vi "Compute 1-Exp Gate Array v2.vi"(8 "Error In":errorcluster, 9 "Gates Definitions":T3={"First Gate: t1"=0.0, "Gate Width: W"=0.0, "Gate Step: d"=0.0, "# Gates: G"=0.0, "Use Gate Center"=FALSE, "Frames/Image: F"=50, "Gates/Frame: L"=0, "Bits/Frame: q"=0, "Multiplicity: p"=0, "Gate Type"=enum."Square", "Gate Edge s"=4.0, "Gate Top Slope"=4.0, "Reversed Sawtooth?"=FALSE, "Computation"=FALSE, "User-defined Gate"={"X Array"=[], "Y Array"=[]}, "Tolerance"=50.0, "Integration"=enum."Item 0", "# Steps"=50.0, "Type of User-defined Function"=enum."Gate"}, 11 "Decay Definition":T1={"offset: t0"=0.0, "period: T"=0.0, "lifetime: tau"=0.0, "Incident Signal: I"=0.5, "Normalized Decays"=FALSE, "IRF Model"=enum."Dirac", "IRF Parameter 1"=0.0}) -> (0 "Error Out":errorcluster, 1 "Gate Image Array":ext[](array[numeric]), 3 "t Array":ext[](array[numeric]), 4 "Small Gate Values?":bool, 6 "CPU (s)":dbl)   [LabVIEW 2019]
uses:
  Gate Definitions.ctl
  Gate Type.ctl
  XY Plot Data.ctl
  Decay Definiton.ctl
  IRF Model.ctl
  Photon-Counting Saturation Parameters.ctl
  Linear Ramp End Options.ctl
  Gate & Decay Parameters.ctl
  <vilib>/Analysis/2dsp.llb/Integral Method.ctl
  <vilib>/Utility/High Resolution Relative Seconds.vi
  9dc9122e-8396-4e29-9b52-206296392f6e.vi/00547001-b378-40f2-b110-93d9ac793ed4.vi
  9dc9122e-8396-4e29-9b52-206296392f6e.vi/724eff8e-639b-48e4-a8a7-ae0679ec3008.vi
  09e65239-3f09-4922-a97b-00e12ebb298a.vi/1890a3e4-7c62-4218-b57e-fb16b0242503.vi
  09e65239-3f09-4922-a97b-00e12ebb298a.vi/c3b045bd-7c36-4fc1-8ca3-e82ed1323710.vi
  430a8be0-ec63-490d-ae91-6adec514d333.vi/2230d1ff-c83d-4d4a-9baa-48ca351c5a01.vi
  430a8be0-ec63-490d-ae91-6adec514d333.vi/64cd5ee0-de3b-48e4-a251-9d7fe93364db.vi
  9329e439-e603-4ca8-9979-680bb8b82628.vi/ea36ca11-d45e-4734-8ad6-4c8212e9470a.vi
  9329e439-e603-4ca8-9979-680bb8b82628.vi/e2358c8a-5d5c-4bd7-ba4e-bc581c78cc25.vi
  2b2e435f-01ea-4379-bbb3-bd43ea243b44.vi/87f3088b-8e60-4336-978e-9d71afa4fe14.vi
  2b2e435f-01ea-4379-bbb3-bd43ea243b44.vi/e558c6a5-1956-4c97-b49d-79e0ed7d8e6e.vi
  SEPXP Globals.vi
  <vilib>/ErrorRing/Error Ring.xnode
  <vilib>/Analysis/NI_AALPro.lvlib
panel:
  out "XY Graph":cluster{ext[], ext[]}[](graph)
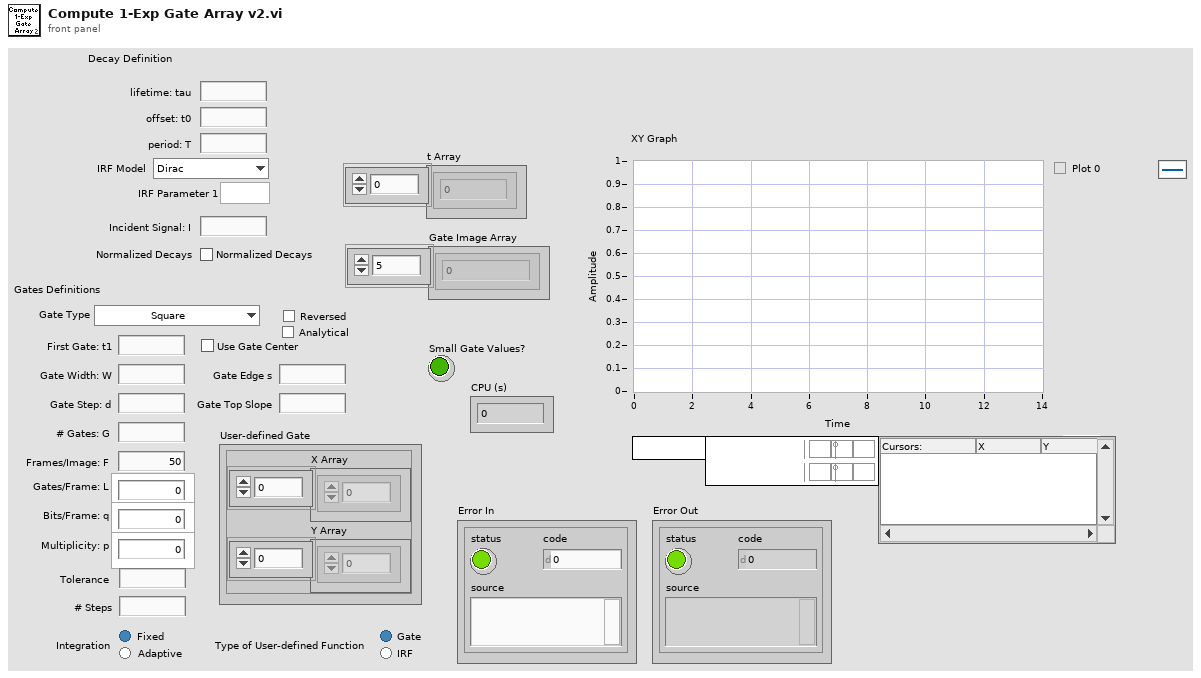
[diagram p1: front panel]
types:
  T1 = typedef "Decay Definiton.ctl" = cluster{"offset: t0":ext, "period: T":ext, "lifetime: tau":ext, "Incident Signal: I":ext, "Normalized Decays":bool, "IRF Model":T2, "IRF Parameter 1":ext}
  T2 = typedef "IRF Model.ctl" = enum16{"Dirac", "Exponential"}
  T3 = typedef "Gate Definitions.ctl" = cluster{"First Gate: t1":ext, "Gate Width: W":ext, "Gate Step: d":ext, "# Gates: G":ext, "Use Gate Center":bool, "Frames/Image: F":i32, "Gates/Frame: L":i32, "Bits/Frame: q":i32, "Multiplicity: p":i32, "Gate Type":T4, "Gate Edge s":ext, "Gate Top Slope":ext, "Reversed Sawtooth?":bool, "Computation":bool, "User-defined Gate":T5, "Tolerance":ext, "Integration":enum32{"Item 0", "Item 1"}, "# Steps":ext, "Type of User-defined Function":enum32{"Gate", "IRF"}}
  T4 = typedef "Gate Type.ctl" = enum16{"Square", "Finite Edge Square", "Finite Edge, Tilted Top Square", "Triangle", "Sawtooth", "User-defined"}
  T5 = typedef "XY Plot Data.ctl" = cluster{"X Array":dbl[], "Y Array":dbl[]}
  T6 = typedef "Photon-Counting Saturation Parameters.ctl" = cluster{"Frames/Image: F":i32, "Gates/Frame: L":i32, "Multiplicity: p":i32, "Bits/Frame: q":i32}
  T7 = typedef "Gate & Decay Parameters.ctl" = cluster{"W":dbl, "T":dbl, "tau":dbl, "t_0":dbl, "Gate Type":T4, "t_i":dbl, "sR":dbl, "sF":dbl, "s":dbl, "Reversed Sawtooth":bool, "IRF Model":T2, "IRF Parameter 1":dbl, "User-defined Gate":T5, "Type of User-defined Function":enum32{"Gate", "IRF"}}
  T8 = typedef "Linear Ramp End Options.ctl" = enum16{"Include Min/Exclude Max", "Exclude Min/Include Max", "Include Both Ends", "Exclude Both Ends"}
  T9 = typedef "NI_AALPro.lvlib/Integral Method.ctl" = i32
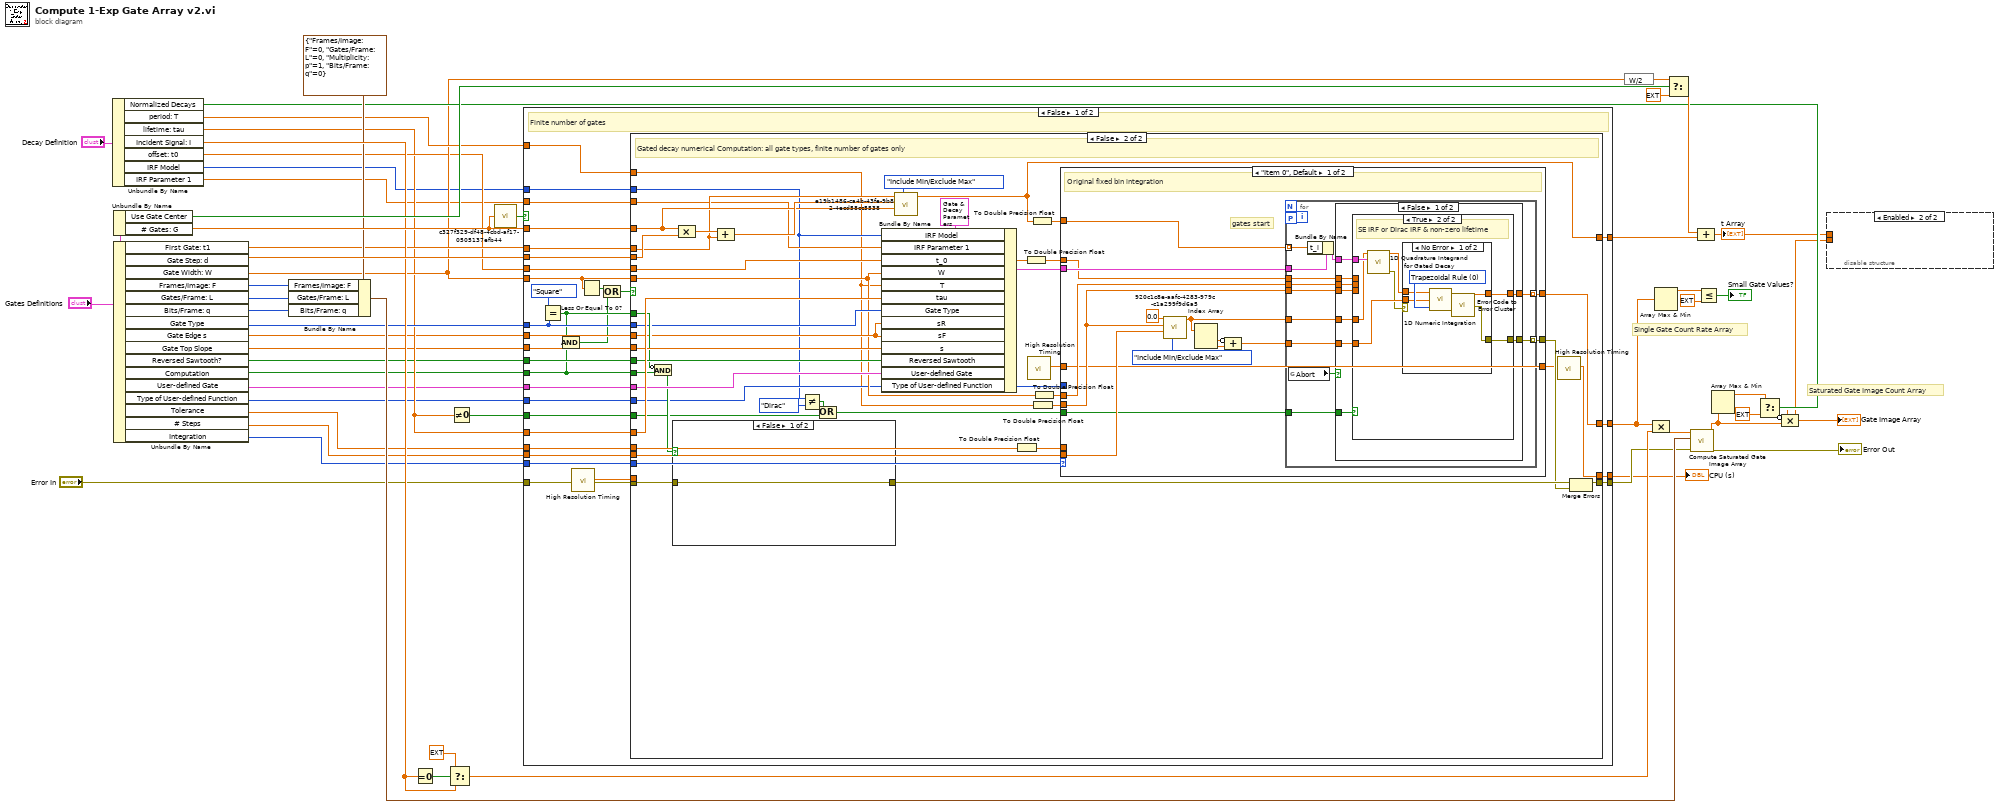
[diagram p0: block diagram]
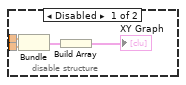
[diagram p2: hidden frame]
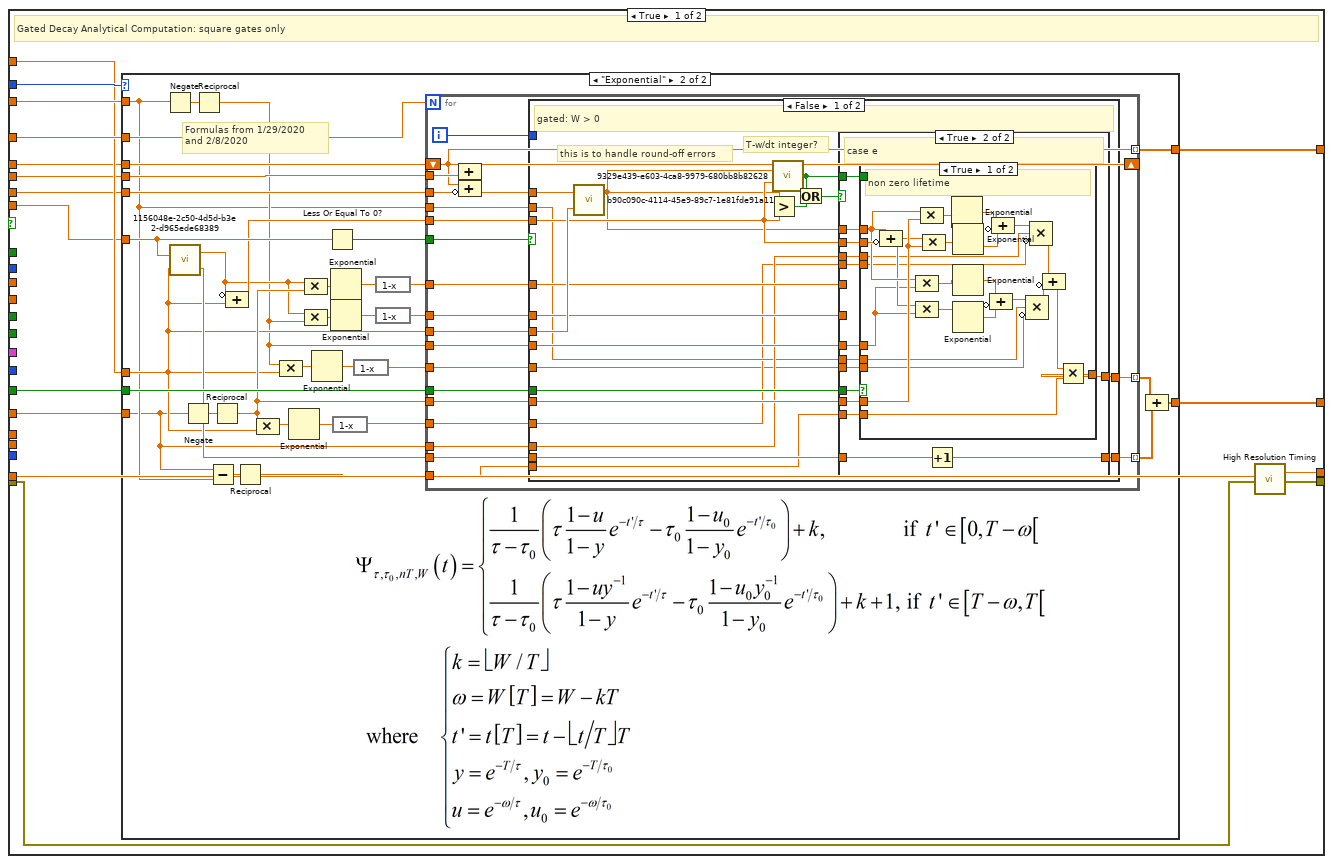
[diagram p3: hidden frame]
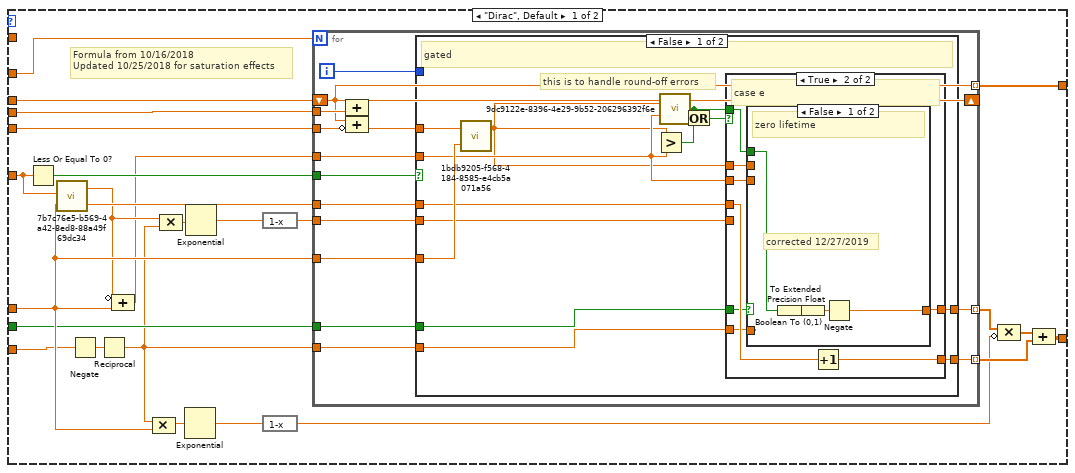
[diagram p4: hidden frame]
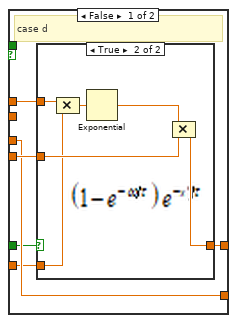
[diagram p5: hidden frame]
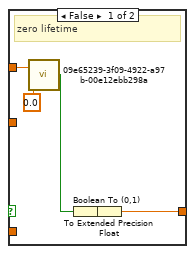
[diagram p6: hidden frame]
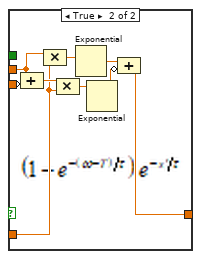
[diagram p7: hidden frame]
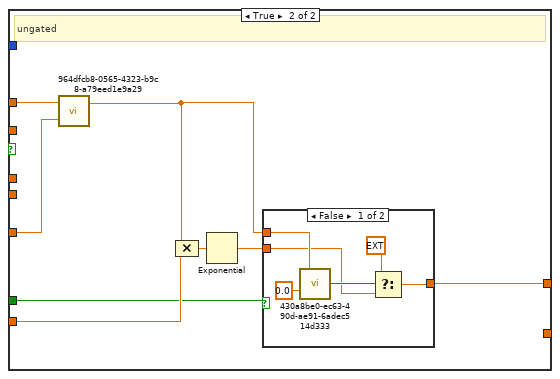
[diagram p8: hidden frame]
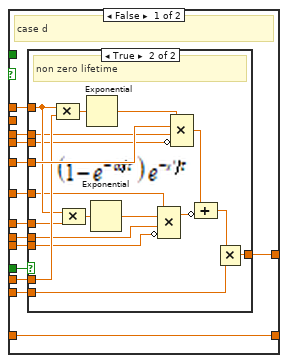
[diagram p10: hidden frame]
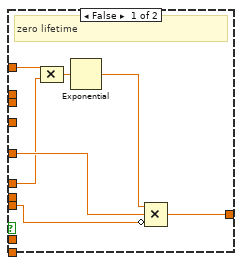
[diagram p11: hidden frame]
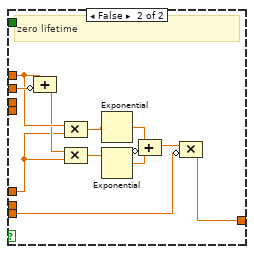
[diagram p12: hidden frame]
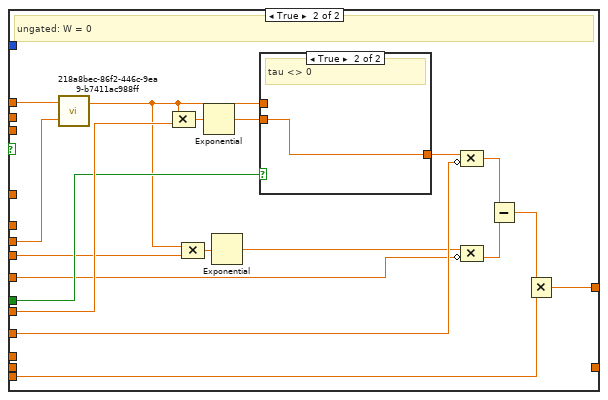
[diagram p13: hidden frame]
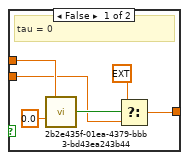
[diagram p14: hidden frame]
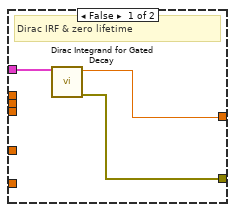
[diagram p15: hidden frame]
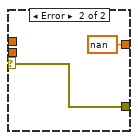
[diagram p16: hidden frame]
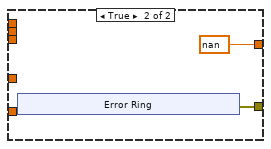
[diagram p17: hidden frame]
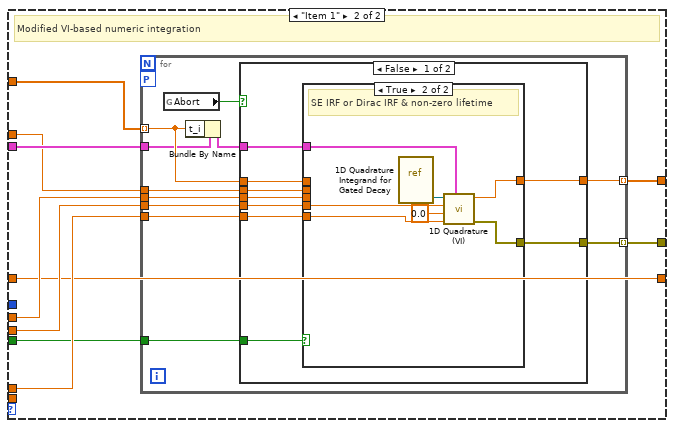
[diagram p18: hidden frame]
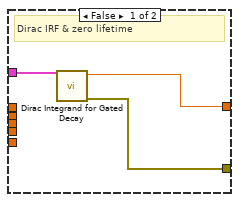
[diagram p19: hidden frame]
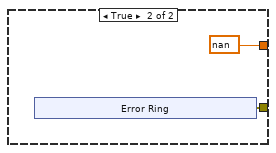
[diagram p20: hidden frame]
diagram:
  # "Saturated Gate Image Count Array"
  # "Single Gate Count Rate Array"
  n1 = Unbundle By Name("Decay Definition") -> ("Normalized Decays"=w33:bool, "period: T"=w29:ext, "lifetime: tau"=w20:ext, "Incident Signal: I"=w42:ext, "offset: t0"=w24:ext, "IRF Model"=w8:T2, "IRF Parameter 1"=w7:ext)
  n2 = Unbundle By Name("Gates Definitions") -> ("Use Gate Center"=w46:bool, "# Gates: G"=w47:ext)
  n3 = Unbundle By Name("Gates Definitions") -> ("First Gate: t1"=w30:ext, "Gate Step: d"=w53:ext, "Gate Width: W"=w25:ext, "Frames/Image: F"=w40:i32, "Gates/Frame: L"=w39:i32, "Bits/Frame: q"=w38:i32, "Gate Type"=w23:T4, "Gate Edge s"=w18:ext, "Gate Top Slope"=w17:ext, "Reversed Sawtooth?"=w13:bool, "Computation"=w9:bool, "User-defined Gate"=w6:T5, "Type of User-defined Function"=w1:enum32{"Gate", "IRF"}, "Tolerance"=w5:ext, "# Steps"=w2:ext, "Integration"=w3:enum32{"Item 0", "Item 1"})
  n4 = Bundle By Name(cluster=T6 {"Frames/Image: F"=0, "Gates/Frame: L"=0, "Multiplicity: p"=1, "Bits/Frame: q"=0} ("Saturation Parameters"), "Frames/Image: F"=w40, "Gates/Frame: L"=w39, "Bits/Frame: q"=w38) -> (w37:T6)
  n5 = Equal To 0?(x=w42) -> (x = 0?=w43:bool)
  n6 = Select(t=ext 1.0, s=w43, f=w42) -> (s? t:f=w44:ext)
  n7 = Not Equal To 0?(x=w20) -> (x != 0?=w19:bool)
  n8 = call "c327f329-df48-4cbd-af17-0505137efb44.vi"("Number"=w47) -> ("Is NaN or Inf?"=w10:bool)  [unwired: 8 in]
  n9 = case shown="False" w10 {
    tunnel: w23 -> [w70 _]
    tunnel: w30 -> [w85 _]
    tunnel: w53 -> [w84 _]
    tunnel: w24 -> [w83 _]
    tunnel: w29 -> [w82 _]
    tunnel: w20 -> [w81 _]
    tunnel: [w80 _] -> w22
    tunnel: [w79 _] -> w21
    tunnel: w19 -> [w78 _]
    tunnel: w18 -> [w77 _]
    tunnel: w17 -> [w76 _]
    tunnel: w13 -> [w75 _]
    tunnel: w47 -> [w74 _]
    tunnel: w25 -> [w62 _]
    tunnel: "Error In" -> [w72 w555]
    tunnel: [w73 w555] -> w11
    tunnel: w9 -> [w65 _]
    tunnel: w8 -> [w69 _]
    tunnel: w7 -> [w68 _]
    tunnel: w6 -> [w67 _]
    tunnel: w5 -> [w66 _]
    tunnel: [w59 _] -> w4
    tunnel: w3 -> [w56 _]
    tunnel: w2 -> [w55 _]
    tunnel: w1 -> [w54 _]
    frame False {
      # "Finite number of gates"
      n10 = Equal?(x=Gate_Type."Square" ("Gate Type"), y=w70) -> (x = y?=w64:bool)
      n11 = Compound Arithmetic op=AND(w64, w65) -> (w61:bool)
      n12 = call "High Resolution Timing.vi"("Error In"=w72) -> ("elapsed (relative) seconds"=w57:dbl, "Error Out"=w58:errorcluster)  [unwired: 16 in, 1 out]
      n13 = Less Or Equal To 0?(x=w62) -> (x <= 0?=w60:bool)
      n14 = Compound Arithmetic op=OR(w60, w61) -> (w63:bool)
      n15 = case shown="False" w63 {
        tunnel: w74 -> [w95 w437]
        tunnel: w85 -> [w89 w434]
        tunnel: w84 -> [w90 w435]
        tunnel: w83 -> [w91 w414]
        tunnel: w62 -> [w92 w410]
        tunnel: w82 -> [w93 w399]
        tunnel: w81 -> [w94 w436]
        tunnel: [w101 w432] -> w79
        tunnel: [w100 w433] -> w80
        tunnel: w78 -> [w99 w415]
        tunnel: w77 -> [_ w412]
        tunnel: w76 -> [_ w431]
        tunnel: w75 -> [_ w430]
        tunnel: [w88 w425] -> w73
        tunnel: w58 -> [w98 w426]
        tunnel: w70 -> [_ w411]
        tunnel: w69 -> [w97 w401]
        tunnel: w68 -> [w96 w429]
        tunnel: w67 -> [_ w428]
        tunnel: w66 -> [_ w427]
        tunnel: w65 -> [_ w423]
        tunnel: w64 -> [_ w422]
        tunnel: [w86 w403] -> w59
        tunnel: w57 -> [w87 _]
        tunnel: w56 -> [_ w416]
        tunnel: w55 -> [_ w413]
        tunnel: w54 -> [_ w409]
        frame True {
          # "Gated Decay Analytical Computation: square gates only"
          n16 = case shown="\"Exponential\"" w97 {
            tunnel: w95 -> [w126 w242]
            tunnel: w89 -> [w125 w241]
            tunnel: w90 -> [w124 w240]
            tunnel: w91 -> [w123 w239]
            tunnel: w92 -> [w122 w238]
            tunnel: w93 -> [w121 w218]
            tunnel: w94 -> [w120 w208]
            tunnel: [w119 w237] -> w101
            tunnel: [w118 w236] -> w100
            tunnel: w99 -> [w117 w235]
            tunnel: w96 -> [_ w209]
            frame "Dirac", Default {
              # "Formula from 10/16/2018\nUpdated 10/25/2018 for saturation effects"
              n17 = Less Or Equal To 0?(x=w122) -> (x <= 0?=w106:bool)
              n18 = call "7b7c76e5-b569-4a42-8ed8-88a49f69dc34.vi"("y"=w121, "x"=w122) -> ("E(x/y)"=w109:ext, "x - E(x/y)y"=w105:ext)
              n19 = Negate(x=w120) -> (-x=w114:ext)
              n20 = Reciprocal(x=w114) -> (1/x=w104:ext)
              n21 = Compound Arithmetic op=ADD(invert w105, w121) -> (w102:ext)
              n22 = Compound Arithmetic op=MULTIPLY(w104, w121) -> (w113:ext)
              n23 = Compound Arithmetic op=MULTIPLY(w105, w104) -> (w112:ext)
              n24 = Exponential(1:w113) -> (0:w108:ext)
              n25 = Exponential(1:w112) -> (0:w111:ext)
              n26 = expression code="1-x"(w111) -> (w110:ext)
              n27 = expression code="1-x"(w108) -> (w107:ext)
              n28 = for {
                N: w126 -> [_]
                tunnel: w124 -> [w141]
                tunnel: w123 -> [w139]
                tunnel: w121 -> [w137]
                tunnel: w104 -> [w136]
                shift-right: [w140] -> _
                shift-left: w125 -> [w132]
                tunnel: [w132] -> w119 mode=indexing
                tunnel: w110 -> [w135]
                tunnel: w109 -> [w134]
                tunnel: [w128] -> w103 mode=indexing
                tunnel: [w133] -> w116 mode=indexing
                tunnel: w106 -> [w131]
                tunnel: w102 -> [w130]
                tunnel: w117 -> [w129]
                i -> [w127]
                n29 = Compound Arithmetic op=ADD(w132, w141) -> (w140:ext)
                n30 = Compound Arithmetic op=ADD(w132, invert w139) -> (w138:ext)
                n31 = case shown="False" w131 {
                  tunnel: w138 -> [w154 w200]
                  tunnel: w137 -> [w153 w199]
                  tunnel: w136 -> [w147 w198]
                  tunnel: w135 -> [w152 _]
                  tunnel: [w151 w196] -> w128
                  tunnel: w134 -> [w150 _]
                  tunnel: [w149 _] -> w133
                  tunnel: w130 -> [w145 _]
                  tunnel: w129 -> [w146 w193]
                  tunnel: w127 -> [_ _]
                  frame False {
                    # "this is to handle round-off errors"
                    # "gated"
                    n32 = call "1bdb9205-f568-4184-8585-e4cb5a071a56.vi"("y"=w153, "x"=w154) -> ("x - E(x/y)y"=w142:ext)  [unwired: 1 out]
                    n33 = Greater?(x=w142, y=w145) -> (0:w148:bool)
                    n34 = call "9dc9122e-8396-4e29-9b52-206296392f6e.vi"("X"=w142, "Y"=w145) -> ("X ~= Y?"=w144:bool)  [unwired: 13 in]
                    n35 = Or(x=w144, y=w148) -> (x .or. y?=w143:bool)
                    n36 = case shown="True" w143 {
                      tunnel: w152 -> [w160 _]
                      tunnel: [w159 w175] -> w151
                      tunnel: w150 -> [w158 w179]
                      tunnel: [w158 w178] -> w149
                      tunnel: w142 -> [w157 w177]
                      tunnel: w147 -> [w156 w176]
                      tunnel: w145 -> [_ w174]
                      tunnel: w146 -> [w155 w173]
                      tunnel: w144 -> [_ w172]
                      frame False {
                        # "case d"
                        n37 = case shown="True" w155 {
                          tunnel: w160 -> [_ w171]
                          tunnel: [w164 w170] -> w159
                          tunnel: w157 -> [w163 w168]
                          tunnel: w156 -> [_ w167]
                          frame False {
                            # "zero lifetime"
                            n38 = call "09e65239-3f09-4922-a97b-00e12ebb298a.vi"("X"=w163, "Y"=0.0) -> ("X ~= Y?"=w161:bool)  [unwired: 13 in]
                            n39 = Boolean To (0,1)(Boolean=w161) -> (0, 1=w165:i16)
                            n40 = To Extended Precision Float(1:w165) -> (0:w164:ext)
                          }
                          frame True {
                            n41 = Compound Arithmetic op=MULTIPLY(w168, w167) -> (w169:ext)
                            n42 = Exponential(1:w169) -> (0:w166:ext)
                            n43 = Compound Arithmetic op=MULTIPLY(w166, w171) -> (w170:ext)
                          }
                        }
                      }
                      frame True {
                        # "case e"
                        n44 = case shown="False" w173 {
                          tunnel: w177 -> [_ w190]
                          tunnel: w176 -> [_ w189]
                          tunnel: [w181 w185] -> w175
                          tunnel: w174 -> [_ w184]
                          tunnel: w172 -> [w180 _]
                          frame False {
                            # "corrected 12/27/2019"
                            # "zero lifetime"
                            n45 = Boolean To (0,1)(Boolean=w180) -> (0, 1=w183:i16)
                            n46 = To Extended Precision Float(1:w183) -> (0:w182:ext)
                            n47 = Negate(x=w182) -> (-x=w181:ext)
                          }
                          frame True {
                            n48 = Compound Arithmetic op=ADD(w190, invert w184) -> (w192:ext)
                            n49 = Compound Arithmetic op=MULTIPLY(w190, w189) -> (w188:ext)
                            n50 = Compound Arithmetic op=MULTIPLY(w192, w189) -> (w191:ext)
                            n51 = Exponential(1:w188) -> (0:w187:ext)
                            n52 = Exponential(1:w191) -> (0:w186:ext)
                            n53 = Compound Arithmetic op=ADD(w187, invert w186) -> (w185:ext)
                          }
                        }
                        n54 = Increment(x=w179) -> (x+1=w178:ext)
                      }
                    }
                  }
                  frame True {
                    # "ungated"
                    n55 = call "964dfcb8-0565-4323-b9c8-a79eed1e9a29.vi"("y"=w199, "x"=w200) -> ("x - E(x/y)y"=w195:ext)  [unwired: 1 out]
                    n56 = Compound Arithmetic op=MULTIPLY(w195, w198) -> (w197:ext)
                    n57 = Exponential(1:w197) -> (0:w194:ext)
                    n58 = case shown="False" w193 {
                      tunnel: [w206 w207] -> w196
                      tunnel: w195 -> [w205 _]
                      tunnel: w194 -> [w201 w207]
                      frame False {
                        n59 = call "430a8be0-ec63-490d-ae91-6adec514d333.vi"("X"=w205, "Y"=0.0) -> ("X ~= Y?"=w203:bool)  [unwired: 13 in]
                        n60 = Select(t=ext 1.0 ("f"), s=w203, f=w201) -> (s? t:f=w206:ext)
                      }
                      frame True {
                      }
                    }
                  }
                }
              }
              n61 = Compound Arithmetic op=MULTIPLY(w103, invert w107) -> (w115:ext[])
              n62 = Compound Arithmetic op=ADD(w115, w116) -> (w118:ext[])
            }
            frame "Exponential" {
              # "Formulas from 1/29/2020\nand 2/8/2020"
              n63 = Negate(x=w209) -> (-x=w223:ext)
              n64 = call "1156048e-2c50-4d5d-b3e2-d965ede68389.vi"("y"=w218, "x"=w238) -> ("E(x/y)"=w228:ext, "x - E(x/y)y"=w214:ext)
              n65 = Negate(x=w208) -> (-x=w233:ext)
              n66 = Reciprocal(x=w223) -> (1/x=w213:ext)
              n67 = Subtract(x=w208, y=w209) -> (x-y=w211:ext)
              n68 = Reciprocal(x=w233) -> (1/x=w225:ext)
              n69 = Compound Arithmetic op=ADD(invert w214, w218) -> (w224:ext)
              n70 = Reciprocal(x=w211) -> (1/x=w210:ext)
              n71 = Compound Arithmetic op=MULTIPLY(w225, w218) -> (w232:ext)
              n72 = Compound Arithmetic op=MULTIPLY(w213, w218) -> (w219:ext)
              n73 = Exponential(1:w232) -> (0:w227:ext)
              n74 = Compound Arithmetic op=MULTIPLY(w214, w225) -> (w231:ext)
              n75 = Compound Arithmetic op=MULTIPLY(w214, w213) -> (w215:ext)
              n76 = Exponential(1:w219) -> (0:w220:ext)
              n77 = Less Or Equal To 0?(x=w238) -> (x <= 0?=w226:bool)
              n78 = Exponential(1:w231) -> (0:w230:ext)
              n79 = Exponential(1:w215) -> (0:w216:ext)
              n80 = expression code="1-x"(w227) -> (w222:ext)
              n81 = expression code="1-x"(w220) -> (w217:ext)
              n82 = expression code="1-x"(w230) -> (w229:ext)
              n83 = expression code="1-x"(w216) -> (w212:ext)
              n84 = for {
                N: w242 -> [_]
                tunnel: w240 -> [w264]
                tunnel: w239 -> [w262]
                tunnel: w218 -> [w260]
                tunnel: w225 -> [w259]
                shift-right: [w263] -> _
                shift-left: w241 -> [w256]
                tunnel: [w256] -> w237 mode=indexing
                tunnel: w229 -> [w258]
                tunnel: w228 -> [w243]
                tunnel: [w245] -> w221 mode=indexing
                tunnel: [w257] -> w234 mode=indexing
                tunnel: w226 -> [w255]
                tunnel: w224 -> [w254]
                tunnel: w235 -> [w253]
                tunnel: w213 -> [w251]
                tunnel: w222 -> [w246]
                tunnel: w217 -> [w250]
                tunnel: w212 -> [w249]
                tunnel: w210 -> [w244]
                tunnel: w209 -> [w248]
                tunnel: w208 -> [w247]
                i -> [w252]
                n85 = Compound Arithmetic op=ADD(w256, w264) -> (w263:ext)
                n86 = Compound Arithmetic op=ADD(w256, invert w262) -> (w261:ext)
                n87 = case shown="False" w255 {
                  tunnel: w261 -> [w284 w389]
                  tunnel: w260 -> [w283 w388]
                  tunnel: w259 -> [w278 w387]
                  tunnel: w258 -> [w282 _]
                  tunnel: w243 -> [w281 _]
                  tunnel: [w280 _] -> w257
                  tunnel: w254 -> [w276 _]
                  tunnel: w253 -> [w277 w384]
                  tunnel: w252 -> [_ _]
                  tunnel: w251 -> [w272 w380]
                  tunnel: w250 -> [w266 w377]
                  tunnel: w249 -> [w271 _]
                  tunnel: w248 -> [w269 _]
                  tunnel: w247 -> [w270 _]
                  tunnel: w246 -> [w268 w382]
                  tunnel: [w267 w372] -> w245
                  tunnel: w244 -> [w265 w373]
                  frame False {
                    # "T-w/dt integer?"
                    # "this is to handle round-off errors"
                    # "gated: W > 0"
                    n88 = call "b90c090c-4114-45e9-89c7-1e81fde91a11.vi"("y"=w283, "x"=w284) -> ("x - E(x/y)y"=w273:ext)  [unwired: 1 out]
                    n89 = Greater?(x=w273, y=w276) -> (0:w279:bool)
                    n90 = call "9329e439-e603-4ca8-9979-680bb8b82628.vi"("X"=w273, "Y"=w276) -> ("X ~= Y?"=w275:bool)  [unwired: 13 in]
                    n91 = Or(x=w275, y=w279) -> (x .or. y?=w274:bool)
                    n92 = case shown="True" w274 {
                      tunnel: w282 -> [w297 _]
                      tunnel: [w296 w332] -> w267
                      tunnel: w281 -> [w295 w336]
                      tunnel: [w295 w335] -> w280
                      tunnel: w273 -> [w294 w334]
                      tunnel: w278 -> [w293 w333]
                      tunnel: w276 -> [_ w331]
                      tunnel: w277 -> [w292 w330]
                      tunnel: w275 -> [_ w329]
                      tunnel: w272 -> [w291 w328]
                      tunnel: w271 -> [w290 _]
                      tunnel: w270 -> [w289 w327]
                      tunnel: w269 -> [w288 w326]
                      tunnel: w268 -> [w287 w325]
                      tunnel: w266 -> [w286 w324]
                      tunnel: w265 -> [w285 w323]
                      frame False {
                        # "case d"
                        n93 = case shown="True" w292 {
                          tunnel: w297 -> [_ w322]
                          tunnel: [w302 w306] -> w296
                          tunnel: w294 -> [w300 w317]
                          tunnel: w293 -> [_ w319]
                          tunnel: w291 -> [w299 w316]
                          tunnel: w290 -> [w304 w314]
                          tunnel: w289 -> [_ w312]
                          tunnel: w288 -> [_ w311]
                          tunnel: w287 -> [_ w310]
                          tunnel: w286 -> [w303 w309]
                          tunnel: w285 -> [_ w305]
                          frame False {
                            # "zero lifetime"
                            n94 = Compound Arithmetic op=MULTIPLY(w300, w299) -> (w301:ext)
                            n95 = Exponential(1:w301) -> (0:w298:ext)
                            n96 = Compound Arithmetic op=MULTIPLY(w298, w304, invert w303) -> (w302:ext)
                          }
                          frame True {
                            # "non zero lifetime"
                            n97 = Compound Arithmetic op=MULTIPLY(w317, w319) -> (w320:ext)
                            n98 = Compound Arithmetic op=MULTIPLY(w317, w316) -> (w315:ext)
                            n99 = Exponential(1:w320) -> (0:w318:ext)
                            n100 = Exponential(1:w315) -> (0:w313:ext)
                            n101 = Compound Arithmetic op=MULTIPLY(w314, w313, w311, invert w309) -> (w307:ext)
                            n102 = Compound Arithmetic op=MULTIPLY(w318, w322, w312, invert w310) -> (w321:ext)
                            n103 = Compound Arithmetic op=ADD(w321, invert w307) -> (w308:ext)
                            n104 = Multiply(x=w308, y=w305) -> (x*y=w306:ext)
                          }
                        }
                      }
                      frame True {
                        # "case e"
                        n105 = case shown="True" w330 {
                          tunnel: w334 -> [w353 w370]
                          tunnel: w333 -> [w359 _]
                          tunnel: [w338 w361] -> w332
                          tunnel: w331 -> [w354 w371]
                          tunnel: w329 -> [_ _]
                          tunnel: w328 -> [w351 w368]
                          tunnel: w327 -> [w345 _]
                          tunnel: w326 -> [w343 _]
                          tunnel: w325 -> [w342 _]
                          tunnel: w324 -> [w341 w362]
                          tunnel: w323 -> [w337 _]
                          frame True {
                            # "non zero lifetime"
                            n106 = Compound Arithmetic op=ADD(w353, invert w354) -> (w352:ext)
                            n107 = Compound Arithmetic op=MULTIPLY(w353, w351) -> (w350:ext)
                            n108 = Compound Arithmetic op=MULTIPLY(w352, w351) -> (w349:ext)
                            n109 = Compound Arithmetic op=MULTIPLY(w353, w359) -> (w358:ext)
                            n110 = Compound Arithmetic op=MULTIPLY(w352, w359) -> (w360:ext)
                            n111 = Exponential(1:w358) -> (0:w357:ext)
                            n112 = Exponential(1:w360) -> (0:w356:ext)
                            n113 = Exponential(1:w350) -> (0:w348:ext)
                            n114 = Exponential(1:w349) -> (0:w347:ext)
                            n115 = Compound Arithmetic op=ADD(w348, invert w347) -> (w344:ext)
                            n116 = Compound Arithmetic op=ADD(w357, invert w356) -> (w355:ext)
                            n117 = Compound Arithmetic op=MULTIPLY(w344, w343, invert w341) -> (w339:ext)
                            n118 = Compound Arithmetic op=MULTIPLY(w355, w345, invert w342) -> (w346:ext)
                            n119 = Compound Arithmetic op=ADD(w346, invert w339) -> (w340:ext)
                            n120 = Multiply(x=w340, y=w337) -> (x*y=w338:ext)
                          }
                          frame False {
                            # "zero lifetime"
                            n121 = Compound Arithmetic op=ADD(w370, invert w371) -> (w369:ext)
                            n122 = Compound Arithmetic op=MULTIPLY(w370, w368) -> (w367:ext)
                            n123 = Compound Arithmetic op=MULTIPLY(w369, w368) -> (w366:ext)
                            n124 = Exponential(1:w367) -> (0:w365:ext)
                            n125 = Exponential(1:w366) -> (0:w364:ext)
                            n126 = Compound Arithmetic op=ADD(w365, invert w364) -> (w363:ext)
                            n127 = Compound Arithmetic op=MULTIPLY(w363, invert w362) -> (w361:ext)
                          }
                        }
                        n128 = Increment(x=w336) -> (x+1=w335:ext)
                      }
                    }
                  }
                  frame True {
                    # "ungated: W = 0"
                    n129 = call "218a8bec-86f2-446c-9ea9-b7411ac988ff.vi"("y"=w388, "x"=w389) -> ("x - E(x/y)y"=w381:ext)  [unwired: 1 out]
                    n130 = Compound Arithmetic op=MULTIPLY(w381, w387) -> (w386:ext)
                    n131 = Compound Arithmetic op=MULTIPLY(w381, w380) -> (w379:ext)
                    n132 = Exponential(1:w386) -> (0:w385:ext)
                    n133 = Exponential(1:w379) -> (0:w378:ext)
                    n134 = case shown="True" w384 {
                      tunnel: [w395 w396] -> w383
                      tunnel: w381 -> [w394 _]
                      tunnel: w385 -> [w390 w396]
                      frame False {
                        # "tau = 0"
                        n135 = call "2b2e435f-01ea-4379-bbb3-bd43ea243b44.vi"("X"=w394, "Y"=0.0) -> ("X ~= Y?"=w392:bool)  [unwired: 13 in]
                        n136 = Select(t=ext 1.0 ("f"), s=w392, f=w390) -> (s? t:f=w395:ext)
                      }
                      frame True {
                        # "tau <> 0"
                      }
                    }
                    n137 = Compound Arithmetic op=MULTIPLY(w383, invert w382) -> (w376:ext)
                    n138 = Compound Arithmetic op=MULTIPLY(w378, invert w377) -> (w375:ext)
                    n139 = Subtract(x=w376, y=w375) -> (x-y=w374:ext)
                    n140 = Multiply(x=w374, y=w373) -> (x*y=w372:ext)
                  }
                }
              }
              n141 = Compound Arithmetic op=ADD(w221, w234) -> (w236:ext[])
            }
          }
          n142 = call "High Resolution Timing.vi"("relative seconds (NaN)"=w87, "Error In"=w98) -> ("elapsed (relative) seconds"=w86:dbl, "Error Out"=w88:errorcluster)  [unwired: 15 in, 1 out]
        }
        frame False {
          # "Gated decay numerical Computation: all gate types, finite number of gates only"
          n143 = Compound Arithmetic op=AND(invert w422, w423) -> (w421:bool)
          n144 = case shown="False" w421 {
            selector: w421 -> [_ w549]
            tunnel: w426 -> [w548 w553]
            tunnel: [w548 w551] -> w424
            frame False {
            }
            frame True {
              # "Analytical Calculation requested for non-square gate"
              n145 = call <vilib>:"Error Cluster From Error Code.vi"("is warning? (False)"=w549, "error in (no error)"=w553, "error message (\"\")"="Analytical computation not avalaible for non square gates: using numerical computation instead..." ("message"), "error code (0)"=1) -> ("error out"=w551:errorcluster)  [unwired: 5 in]
            }
          }
          n146 = Compound Arithmetic op=MULTIPLY(w437, w435) -> (w440:ext)
          n147 = Compound Arithmetic op=ADD(w440, w434) -> (w439:ext)
          n148 = Not Equal?(x=w401, y=IRF_Model."Dirac" ("IRF Model")) -> (x != y?=w398:bool)
          n149 = Compound Arithmetic op=OR(w398, w415) -> (w397:bool)
          n150 = Bundle By Name(cluster=T7 {"W"=0.0, "T"=0.0, "tau"=0.0, "t_0"=0.0, "Gate Type"=enum."Square", "t_i"=0.0, "sR"=0.0, "sF"=0.0, "s"=0.0, "Reversed Sawtooth"=FALSE, "IRF Model"=enum."Dirac", "IRF Parameter 1"=0.0, "User-defined Gate"={"X Array"=[], "Y Array"=[]}, "Type of User-defined Function"=enum."Gate"} ("Gate & Decay Parameters"), "IRF Model"=w401, "IRF Parameter 1"=w429, "t_0"=w414, "W"=w410, "T"=w399, "tau"=w436, "Gate Type"=w411, "sR"=w412, "sF"=w412, "s"=w431, "Reversed Sawtooth"=w430, "User-defined Gate"=w428, "Type of User-defined Function"=w409) -> (w419:T7)
          n151 = call "e19b1486-ca4b-43fe-9b82-4ecd58cc5538.vi"("Options"=Linear_Ramp_End_Options."Include Min/Exclude Max", "# Steps (1)"=w437, "End (1)"=w439, "Start (0)"=w434) -> ("Ramp"=w432:ext[])  [unwired: 6 in, 1 out]
          n152 = To Double Precision Float(number=w427) -> (double precision float=w405:dbl)
          n153 = To Double Precision Float(number=w414) -> (double precision float=w408:dbl)
          n154 = call "High Resolution Timing.vi"() -> ("elapsed (relative) seconds"=w404:dbl)  [unwired: 17 in, 2 out]
          n155 = To Double Precision Float(number=w432) -> (double precision float=w417:dbl[])
          n156 = To Double Precision Float(number=w399) -> (double precision float=w406:dbl)
          n157 = To Double Precision Float(number=w410) -> (double precision float=w407:dbl)
          n158 = case shown="\"Item 0\", Default" w416 {
            tunnel: [w456 w508] -> w433
            tunnel: w405 -> [_ w506]
            tunnel: w419 -> [w455 w509]
            tunnel: [w447 w507] -> w418
            tunnel: w417 -> [w448 w511]
            tunnel: w407 -> [w443 w510]
            tunnel: w406 -> [w444 w505]
            tunnel: w408 -> [w446 w504]
            tunnel: w413 -> [w445 _]
            tunnel: w409 -> [_ _]
            tunnel: w404 -> [w442 w503]
            tunnel: [w442 w503] -> w402
            tunnel: w397 -> [w441 w502]
            frame "Item 0", Default {
              # "gates start"
              # "Original fixed bin integration"
              n159 = call "920c1c8e-aafc-4283-979c-c1a299f9d6a5.vi"("Options"=Linear_Ramp_End_Options."Include Min/Exclude Max", "# Steps (1)"=w445, "End (1)"=w444, "Start (0)"=0.0) -> ("Ramp"=w451:ext[])  [unwired: 6 in, 1 out]
              n160 = Index Array(array=w451) -> (element #1=w452:ext, element #2=w450:ext)  [unwired: 2 in]
              n161 = Compound Arithmetic op=ADD(invert w452, w450) -> (w449:ext)
              n162 = for {
                tunnel: w455 -> [w468]
                tunnel: w448 -> [w462] mode=indexing
                tunnel: w451 -> [w466]
                tunnel: [w465] -> w456 mode=indexing
                tunnel: w449 -> [w464]
                workers-P: _ -> [_]
                tunnel: [w463] -> w447 mode=indexing
                tunnel: w446 -> [w461]
                tunnel: w443 -> [w460]
                tunnel: w444 -> [w459]
                tunnel: w441 -> [w457]
                n163 = global read "SEPXP Globals.vi" "Abort"() -> (w458:bool)
                n164 = Bundle By Name(cluster=w468, "t_i"=w462) -> (w467:T7)
                n165 = case shown="False" w458 {
                  tunnel: w467 -> [w477 _]
                  tunnel: w466 -> [w476 _]
                  tunnel: [w475 nan ("result")] -> w465
                  tunnel: w464 -> [w474 _]
                  tunnel: [w473 w496] -> w463
                  tunnel: w461 -> [w472 _]
                  tunnel: w460 -> [w471 _]
                  tunnel: w459 -> [w470 _]
                  tunnel: w457 -> [w469 _]
                  frame False {
                    n166 = case shown="True" w469 {
                      tunnel: w477 -> [w480 w487]
                      tunnel: w476 -> [_ w485]
                      tunnel: [w479 w484] -> w475
                      tunnel: w474 -> [_ w483]
                      tunnel: [w478 w481] -> w473
                      tunnel: w472 -> [_ _]
                      tunnel: w471 -> [_ _]
                      tunnel: w470 -> [_ _]
                      frame False {
                        # "Dirac IRF & zero lifetime"
                        n167 = call "Dirac Integrand for Gated Decay.vi"("data"=w480) -> ("Error Out"=w478:errorcluster, "F(X)"=w479:dbl)  [unwired: 9 in]
                      }
                      frame True {
                        # "SE IRF or Dirac IRF & non-zero lifetime"
                        n168 = call "1D Quadrature Integrand for Gated Decay.vi"("data"=w487, "X"=w485) -> ("Error Out"=w482:errorcluster, "F(X)"=w486:dbl[])  [unwired: 8 in]
                        n169 = case shown="No Error" w482 {
                          selector: w482 -> [_ w495]
                          tunnel: w486 -> [w492 _]
                          tunnel: [w491 nan ("result")] -> w484
                          tunnel: w483 -> [w490 _]
                          tunnel: [w488 w495] -> w481
                          frame No Error {
                            w493 = T9 0 items=["Trapezoidal Rule", "Simpson's Rule", "Simpson's 3/8 Rule", "Bode Rule"] ("integration method")
                            n170 = call <vilib>:"1D Numeric Integration.vi"("integration method"=w493, "dt"=w490, "Input Array"=w492) -> ("error"=w489:i32, "result"=w491:dbl)
                            n171 = call "Error Code to Error Cluster.vi"("Error Code"=w489) -> ("Error Out"=w488:errorcluster)
                          }
                          frame Error {
                          }
                        }
                      }
                    }
                  }
                  frame True {
                    n172 = xnode "Error Ring"() -> ("error out"=w496:errorcluster)
                  }
                }
              }
            }
            frame "Item 1" {
              # "Modified VI-based numeric integration"
              n173 = for {
                tunnel: w511 -> [w516] mode=indexing
                tunnel: w509 -> [w515]
                tunnel: [w522] -> w508 mode=indexing
                workers-P: _ -> [_]
                tunnel: [w519] -> w507 mode=indexing
                tunnel: w506 -> [w521]
                tunnel: w504 -> [w518]
                tunnel: w505 -> [w517]
                tunnel: w510 -> [w513]
                tunnel: w502 -> [w512]
                n174 = global read "SEPXP Globals.vi" "Abort"() -> (w520:bool)
                n175 = Bundle By Name(cluster=w515, "t_i"=w516) -> (w514:T7)
                n176 = case shown="False" w520 {
                  tunnel: w516 -> [w531 _]
                  tunnel: w514 -> [w530 _]
                  tunnel: [w529 nan ("result")] -> w522
                  tunnel: [w528 w542] -> w519
                  tunnel: w521 -> [w527 _]
                  tunnel: w518 -> [w526 _]
                  tunnel: w517 -> [w525 _]
                  tunnel: w513 -> [w524 _]
                  tunnel: w512 -> [w523 _]
                  frame False {
                    n177 = case shown="True" w523 {
                      tunnel: [w533 w541] -> w529
                      tunnel: w530 -> [w534 w540]
                      tunnel: [w532 w539] -> w528
                      tunnel: w527 -> [_ w538]
                      tunnel: w531 -> [_ _]
                      tunnel: w526 -> [_ _]
                      tunnel: w525 -> [_ w536]
                      tunnel: w524 -> [_ _]
                      frame False {
                        # "Dirac IRF & zero lifetime"
                        n178 = call "Dirac Integrand for Gated Decay.vi"("data"=w534) -> ("Error Out"=w532:errorcluster, "F(X)"=w533:dbl)  [unwired: 9 in]
                      }
                      frame True {
                        # "SE IRF or Dirac IRF & non-zero lifetime"
                        n179 = vi-ref "1D Quadrature Integrand for Gated Decay.vi"() -> (w535:refnum<vi>)
                        n180 = call "1D Quadrature (VI).vi"("data"=w540, "tolerance"=w538, "lower limit"=0.0, "upper limit"=w536, "integrand"=w535) -> ("Error Out"=w539:errorcluster, "result"=w541:dbl)  [unwired: 5 in]
                      }
                    }
                  }
                  frame True {
                    n181 = xnode "Error Ring"() -> ("error out"=w542:errorcluster)
                  }
                }
              }
            }
          }
          n182 = call "High Resolution Timing.vi"("relative seconds (NaN)"=w402) -> ("elapsed (relative) seconds"=w403:dbl)  [unwired: 16 in, 2 out]
          n183 = Merge Errors(w424, w418) -> (w425:errorcluster)
        }
      }
    }
    frame True {
      # "Infinite number of gates"
      n184 = One Button Dialog(message="Can't compute an infinite number of gates, unless the gate is square, in which case an analytical approach is used...\nIn all other cases, use a finite number of gates (Settings>>Gates>># Gates).") -> ()  [unwired: 1 in, 1 out]
    }
  }
  "CPU (s)" <- w4
  n185 = expression code="W/2"(w25) -> (w49:ext)
  n186 = Compound Arithmetic op=MULTIPLY(w22, w44) -> (w41:ext[])
  n187 = Array Max & Min(array=w22) -> (max value=w26:ext)  [unwired: 3 out]
  n188 = Select(t=w49, s=w46, f=ext 0.0 ("t")) -> (s? t:f=w51:ext)
  n189 = call "Compute Saturated Gate Image Array.vi"("error in (no error)"=w11, "Saturation Parameters"=w37, "Gate Count Rate Array in"=w41) -> ("error out"=→"Error Out":errorcluster, "Saturated Gate Image Count Array out"=w34:ext[])  [unwired: 7 in]
  n190 = Less Or Equal?(x=w26, y=ext 1.0842021724855044e-19) -> (x <= y?=→"Small Gate Values?":bool)
  n191 = Compound Arithmetic op=ADD(w51, w21) -> (w16:ext[])
  "t Array" <- w16
  n192 = Array Max & Min(array=w34) -> (max value=w15:ext)  [unwired: 3 out]
  n193 = Select(t=w15, s=w33, f=ext 1.0) -> (s? t:f=w32:ext)
  n194 = Compound Arithmetic op=MULTIPLY(invert w32, w34) -> (w14:ext[])
  "Gate Image Array" <- w14
  n195 = disable-structure shown="Enabled" {
    disable-tunnel: w16 -> [w559 _]
    disable-tunnel: w14 -> [w556 _]
    frame Disabled {
      n196 = Bundle(w559, w556) -> (w557:cluster{ext[], ext[]})  [unwired: 1 in]
      n197 = Build Array(w557) -> (→"XY Graph":cluster{ext[], ext[]}[])
    }
    frame Enabled {
    }
  }
